vi "Draw tick on circle.vi"(6 "inner radius":dbl, 7 "outer radius":dbl, 8 "color":u32(colorbox)=16711695, 9 "Shaft Position":cluster{"horizontal":i16, "vertical":i16}, 10 "Motor Position":dbl[unit], 11 "picture in":picture) -> (2 "outer tick":cluster{dbl, dbl}, 3 "picture out":picture)   [LabVIEW 2020]
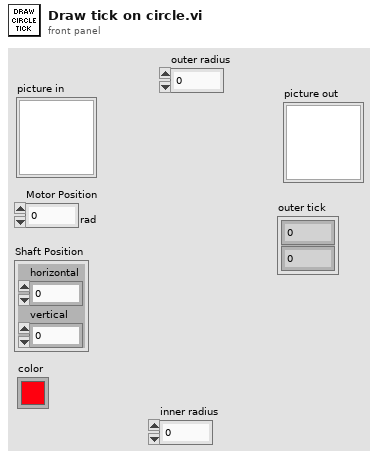
[diagram p1: front panel]
types:
  T1 = cluster{"Width":u16, "Style":enum32{"Solid", "Dash", "Dot", "DashDot", "DashDotDot"}}
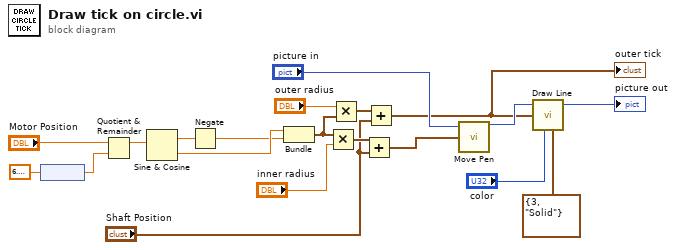
[diagram p0: block diagram]
diagram:
  n1 = node(6.283185307179586) -> (w9:dbl[unit])
  n2 = Quotient & Remainder(x="Motor Position", y=w9) -> (x-y*floor(x/y)=w10:dbl[unit])  [unwired: 1 out]
  n3 = Sine & Cosine(0:w10) -> (1:w11:dbl, 2:w12:dbl)
  n4 = Negate(x=w11) -> (-x=w1:dbl)
  n5 = Bundle(w12, w1) -> (w14:cluster{dbl, dbl})  [unwired: 1 in]
  n6 = Multiply(x=w14, y="inner radius") -> (x*y=w17:cluster{dbl, dbl})
  n7 = Multiply(x="outer radius", y=w14) -> (x*y=w5:cluster{dbl, dbl})
  n8 = Add(x=w17, y="Shaft Position") -> (x+y=w18:cluster{dbl, dbl})
  n9 = Add(x=w5, y="Shaft Position") -> (x+y=w4:cluster{dbl, dbl})
  "outer tick" <- w4
  n10 = call <vilib>:"Move Pen.vi"("new position"=w18, "picture"="picture in") -> ("new picture"=w16:picture)  [unwired: 3 in]
  n11 = call <vilib>:"Draw Line.vi"("picture"=w16, "end point"=w4, "color(black)"="color", "pen"=T1 {"Width"=3, "Style"=enum."Solid"}) -> ("new picture"=→"picture out":picture)  [unwired: 5 in]
